vi "Measurement Type FG.vi"(6 "Action":enum8{"GET", "SET"}(ring), 8 "error in (no error)":errorcluster, 10 "Sample rate (S/s)":u32=500000, 11 "Item Ref":T1 format="%.0x") -> (0 "error out":errorcluster, 2 "Sample rate (S/s)":u32=500000, 3 "Item Ref out":T1=18446744073709551615 format="%.0x")   [LabVIEW 2019, in "Fuel Injector Analysis Addon Shared.lvlib"]
uses:
  Fuel Injector Analysis Addon Shared.lvlib
  <vilib>/NI VeriStand/Custom Device API/Custom Device Item Ref.ctl
  Constants.vi
  <vilib>/NI VeriStand/Custom Device API/Get Item Property (U32).vi
  <vilib>/NI VeriStand/Custom Device API/Set Item Property (U32).vi
  <vilib>/NI VeriStand/Custom Device API/Custom Device API.lvlib
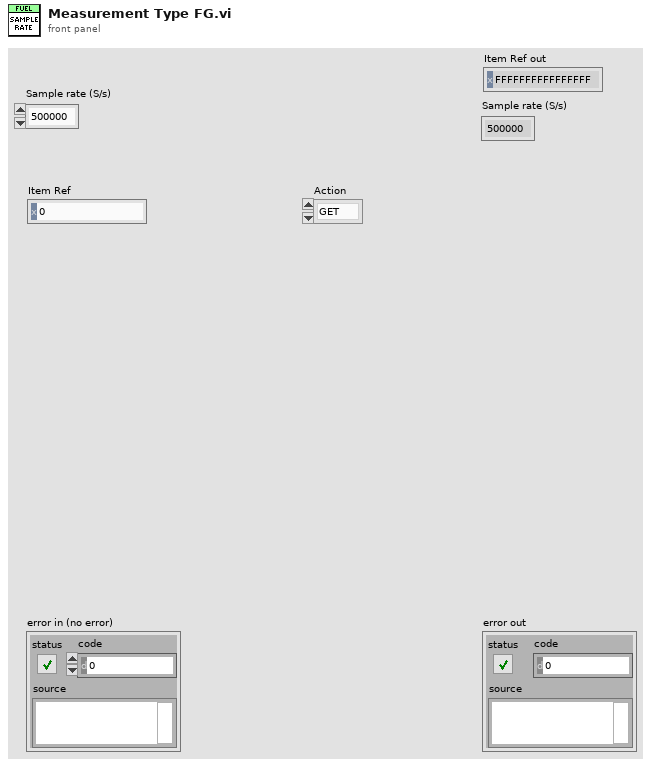
[diagram p1: front panel]
types:
  T1 = typedef "Custom Device API.lvlib/Custom Device Item Ref.ctl" = u64
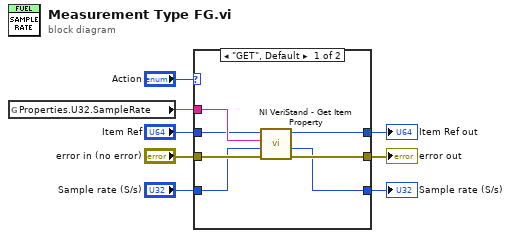
[diagram p0: block diagram]
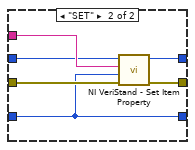
[diagram p2: hidden frame]
diagram:
  n1 = global read "Constants.vi" "Properties.U32.SampleRate"() -> (w2:string)
  n2 = case shown="\"GET\", Default" "Action" {
    tunnel: "error in (no error)" -> [w12 w20]
    tunnel: "Item Ref" -> [w11 w19]
    tunnel: "Sample rate (S/s)" -> [w9 w16]
    tunnel: [w13 w18] -> w4
    tunnel: [w14 w17] -> w7
    tunnel: [w10 w16] -> w1
    tunnel: w2 -> [w15 w21]
    frame "GET", Default {
      n3 = call-poly <vilib>:"NI VeriStand - Get Item Property.vi"("error in (no error)"=w12, "Default Value"=w9, "Property Name"=w15, "Item Ref in"=w11) -> ("error out"=w13:errorcluster, "Value"=w10:u32, "Item Ref out"=w14:T1)  [unwired: 4 in, 1 out]
    }
    frame "SET" {
      n4 = call-poly <vilib>:"NI VeriStand - Set Item Property.vi"("error in (no error)"=w20, "Value"=w16, "Property Name"=w21, "Item Ref in"=w19) -> ("error out"=w18:errorcluster, "Item Ref out"=w17:T1)  [unwired: 5 in, 1 out]
    }
  }
  "error out" <- w4
  "Item Ref out" <- w7
  "Sample rate (S/s)" <- w1
